vi "aa.vi"() -> ()   [LabVIEW 2014]
panel:
  out "x-y":dbl
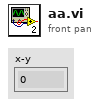
[diagram p1: front panel]
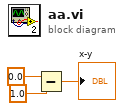
[diagram p0: block diagram]
diagram:
  n1 = Subtract(x=0.0, y=1.0) -> (x-y=→"x-y":dbl)
